vi "简易计算器.vi"() -> ()   [LabVIEW 2018]
panel:
  out "布尔":bool
  out "字符串 3":string
  out "结果":dbl
  out "数字":dbl
  out "字符串 2":string
  out "字符串":string
  in  "簇":T1
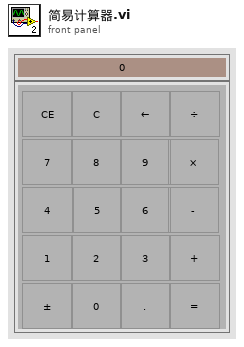
[diagram p1: front panel]
types:
  T1 = cluster{"确定按钮":bool, "确定按钮 2":bool, "确定按钮 3":bool, "确定按钮 4":bool, "确定按钮 5":bool, "确定按钮 6":bool, "确定按钮 7":bool, "确定按钮 8":bool, "确定按钮 9":bool, "确定按钮 10":bool, "确定按钮 17":bool, "确定按钮 18":bool, "确定按钮 19":bool, "确定按钮 20":bool, "确定按钮 16":bool, "确定按钮 15":bool, "确定按钮 14":bool, "确定按钮 13":bool, "确定按钮 12":bool, "确定按钮 11":bool}
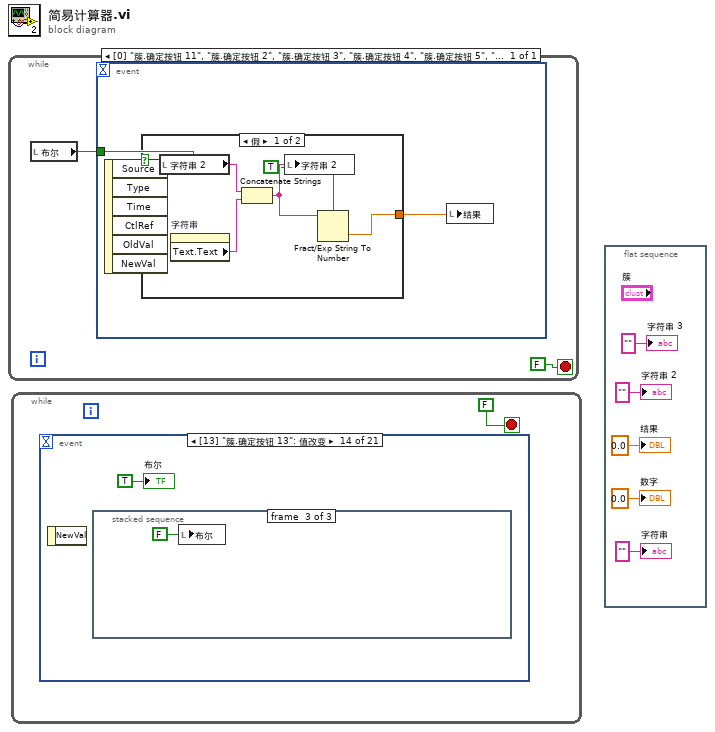
[diagram p0: block diagram]
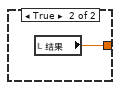
[diagram p2: hidden frame]
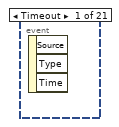
[diagram p3: hidden frame]
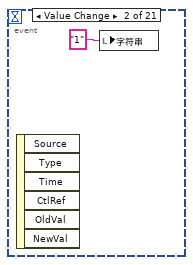
[diagram p4: hidden frame]
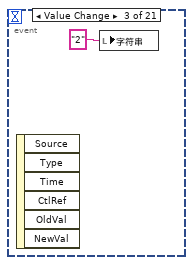
[diagram p5: hidden frame]
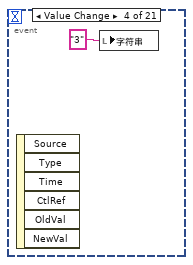
[diagram p6: hidden frame]
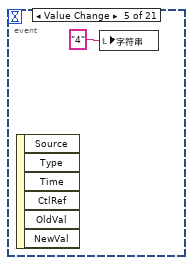
[diagram p7: hidden frame]
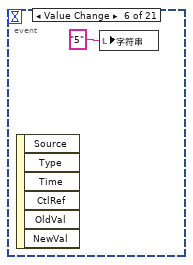
[diagram p8: hidden frame]
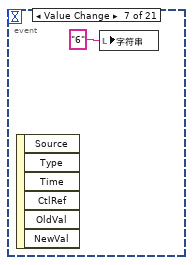
[diagram p9: hidden frame]
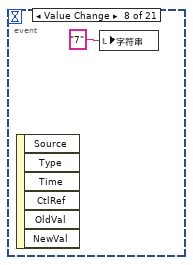
[diagram p10: hidden frame]
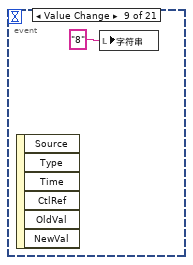
[diagram p11: hidden frame]
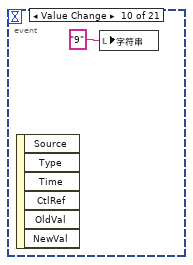
[diagram p12: hidden frame]
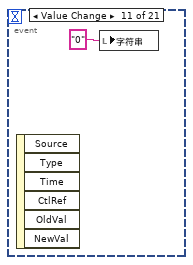
[diagram p13: hidden frame]
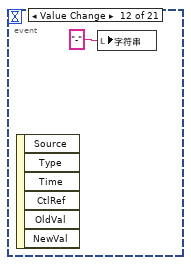
[diagram p14: hidden frame]
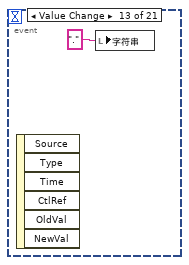
[diagram p15: hidden frame]
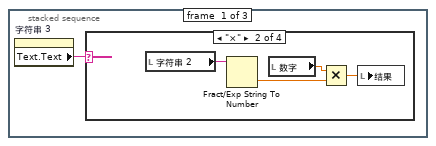
[diagram p16: hidden frame]
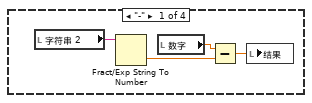
[diagram p17: hidden frame]
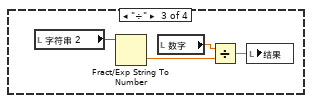
[diagram p18: hidden frame]
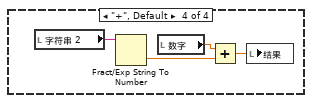
[diagram p19: hidden frame]
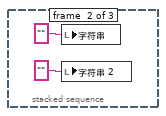
[diagram p20: hidden frame]
diagram:
  n1 = while {
    stop <- FALSE stop-if-true
    n2 = local read "布尔"() -> (w1:bool)
    n3 = event shown="[0] \"簇.确定按钮 11\", \"簇.确定按钮 2\", \"簇.确定按钮 3\", \"簇.确定按钮 4\", \"簇.确定按钮 5\", \"簇.确定按钮 6\", \"簇.确定按钮 7\", \"簇.确定按钮 8\", \"簇.确定按钮 9\", \"簇.确定按钮 10\", \"簇.确定按钮 12\", \"簇.确定按钮\": 值改变" {
      selector: _ -> [_]
      dyn-events: _ -> [_]
      timeout: _ -> [_]
      tunnel: w1 -> [w3]
      event "簇.确定按钮 11", "簇.确定按钮 2", "簇.确定按钮 3", "簇.确定按钮 4", "簇.确定按钮 5", "簇.确定按钮 6", "簇.确定按钮 7", "簇.确定按钮 8", "簇.确定按钮 9", "簇.确定按钮 10", "簇.确定按钮 12", "簇.确定按钮": Value Change {
        n4 = event-data() -> ()  [unwired: 1 in, 6 out]
        n5 = case shown="假" w3 {
          tunnel: [w7 w10] -> w4
          frame False {
            n6 = local read "字符串 2"() -> (w9:string)
            n7 = property on="字符串" class="Str"() -> ("Text.Text"=w6:string)  [unwired: 2 in, 2 out]
            n8 = Concatenate Strings(w9, w6) -> (w8:string)
            n9 = local write "字符串 2"(w8) -> ()
            n10 = Fract/Exp String To Number(use system decimal point (T)=TRUE ("使用系统小数点(T)"), string=w8) -> (number=w7:dbl)  [unwired: 2 in, 1 out]
          }
          frame True {
            n11 = local read "结果"() -> (w10:dbl)
          }
        }
        n12 = local write "结果"(w4) -> ()
      }
    }
  }
  n13 = while {
    stop <- FALSE stop-if-true
    n14 = event shown="[13] \"簇.确定按钮 13\": 值改变" {
      selector: _ -> [_ _ _ _ _ _ _ _ _ _ _ _ _ _ _ _ _ _ _ _ _]
      dyn-events: _ -> [_ _ _ _ _ _ _ _ _ _ _ _ _ _ _ _ _ _ _ _ _]
      timeout: _ -> [_ _ _ _ _ _ _ _ _ _ _ _ _ _ _ _ _ _ _ _ _]
      event Timeout {
        n15 = event-data() -> ()  [unwired: 1 in, 3 out]
      }
      event "簇.确定按钮": Value Change {
        n16 = event-data() -> ()  [unwired: 1 in, 6 out]
        n17 = local write "字符串"("1" ("字符串")) -> ()
      }
      event "簇.确定按钮 2": Value Change {
        n18 = event-data() -> ()  [unwired: 1 in, 6 out]
        n19 = local write "字符串"("2" ("字符串")) -> ()
      }
      event "簇.确定按钮 3": Value Change {
        n20 = event-data() -> ()  [unwired: 1 in, 6 out]
        n21 = local write "字符串"("3" ("字符串")) -> ()
      }
      event "簇.确定按钮 4": Value Change {
        n22 = event-data() -> ()  [unwired: 1 in, 6 out]
        n23 = local write "字符串"("4" ("字符串")) -> ()
      }
      event "簇.确定按钮 5": Value Change {
        n24 = event-data() -> ()  [unwired: 1 in, 6 out]
        n25 = local write "字符串"("5" ("字符串")) -> ()
      }
      event "簇.确定按钮 6": Value Change {
        n26 = event-data() -> ()  [unwired: 1 in, 6 out]
        n27 = local write "字符串"("6" ("字符串")) -> ()
      }
      event "簇.确定按钮 7": Value Change {
        n28 = event-data() -> ()  [unwired: 1 in, 6 out]
        n29 = local write "字符串"("7" ("字符串")) -> ()
      }
      event "簇.确定按钮 8": Value Change {
        n30 = event-data() -> ()  [unwired: 1 in, 6 out]
        n31 = local write "字符串"("8" ("字符串")) -> ()
      }
      event "簇.确定按钮 9": Value Change {
        n32 = event-data() -> ()  [unwired: 1 in, 6 out]
        n33 = local write "字符串"("9" ("字符串")) -> ()
      }
      event "簇.确定按钮 10": Value Change {
        n34 = event-data() -> ()  [unwired: 1 in, 6 out]
        n35 = local write "字符串"("0" ("字符串")) -> ()
      }
      event "簇.确定按钮 11": Value Change {
        n36 = event-data() -> ()  [unwired: 1 in, 6 out]
        n37 = local write "字符串"("-" ("字符串")) -> ()
      }
      event "簇.确定按钮 12": Value Change {
        n38 = event-data() -> ()  [unwired: 1 in, 6 out]
        n39 = local write "字符串"("." ("字符串")) -> ()
      }
      event "簇.确定按钮 13": Value Change {
        n40 = event-data() -> ()  [unwired: 1 in, 1 out]
        n41 = stacked-sequence {
          frame #0 {
            n42 = property on="字符串 3" class="Str"() -> ("Text.Text"=w25:string)  [unwired: 2 in, 2 out]
            n43 = case shown="\"×\"" w25 {
              frame "-" {
                n44 = local read "字符串 2"() -> (w26:string)
                n45 = Fract/Exp String To Number(string=w26) -> (number=w29:dbl)  [unwired: 3 in, 1 out]
                n46 = local read "数字"() -> (w28:dbl)
                n47 = Subtract(x=w28, y=w29) -> (x-y=w27:dbl)
                n48 = local write "结果"(w27) -> ()
              }
              frame "×" {
                n49 = local read "字符串 2"() -> (w30:string)
                n50 = Fract/Exp String To Number(string=w30) -> (number=w33:dbl)  [unwired: 3 in, 1 out]
                n51 = local read "数字"() -> (w32:dbl)
                n52 = Multiply(x=w32, y=w33) -> (x*y=w31:dbl)
                n53 = local write "结果"(w31) -> ()
              }
              frame "÷" {
                n54 = local read "字符串 2"() -> (w34:string)
                n55 = Fract/Exp String To Number(string=w34) -> (number=w37:dbl)  [unwired: 3 in, 1 out]
                n56 = local read "数字"() -> (w36:dbl)
                n57 = Divide(x=w36, y=w37) -> (x/y=w35:dbl)
                n58 = local write "结果"(w35) -> ()
              }
              frame "+", Default {
                n59 = local read "字符串 2"() -> (w40:string)
                n60 = Fract/Exp String To Number(string=w40) -> (number=w39:dbl)  [unwired: 3 in, 1 out]
                n61 = local read "数字"() -> (w41:dbl)
                n62 = Add(x=w41, y=w39) -> (x+y=w38:dbl)
                n63 = local write "结果"(w38) -> ()
              }
            }
          }
          frame #1 {
            n64 = local write "字符串"("" ("字符串")) -> ()
            n65 = local write "字符串 2"("" ("字符串 2")) -> ()
          }
          frame #2 {
            n66 = local write "布尔"(FALSE ("布尔")) -> ()
          }
        }
        "布尔" <- TRUE ("布尔")
      }
      event "簇.确定按钮 14": Value Change {
        n67 = event-data() -> ()  [unwired: 1 in, 6 out]
        n68 = stacked-sequence {
          frame #0 {
            n69 = local read "字符串 2"() -> (w47:string)
            n70 = Fract/Exp String To Number(string=w47) -> (number=w46:dbl)  [unwired: 3 in, 1 out]
            n71 = local write "数字"(w46) -> ()
          }
          frame #1 {
            n72 = local write "字符串"("" ("字符串")) -> ()
            n73 = local write "字符串 2"("" ("字符串 2")) -> ()
          }
        }
        n74 = local write "字符串 3"("+" ("字符串")) -> ()
      }
      event "簇.确定按钮 15": Value Change {
        n75 = event-data() -> ()  [unwired: 1 in, 6 out]
        n76 = stacked-sequence {
          frame #0 {
            n77 = local read "字符串 2"() -> (w52:string)
            n78 = Fract/Exp String To Number(string=w52) -> (number=w51:dbl)  [unwired: 3 in, 1 out]
            n79 = local write "数字"(w51) -> ()
          }
          frame #1 {
            n80 = local write "字符串"("" ("字符串")) -> ()
            n81 = local write "字符串 2"("" ("字符串 2")) -> ()
          }
        }
        n82 = local write "字符串 3"("-" ("字符串")) -> ()
      }
      event "簇.确定按钮 16": Value Change {
        n83 = event-data() -> ()  [unwired: 1 in, 6 out]
        n84 = stacked-sequence {
          frame #0 {
            n85 = local read "字符串 2"() -> (w57:string)
            n86 = Fract/Exp String To Number(string=w57) -> (number=w56:dbl)  [unwired: 3 in, 1 out]
            n87 = local write "数字"(w56) -> ()
          }
          frame #1 {
            n88 = local write "字符串"("" ("字符串")) -> ()
            n89 = local write "字符串 2"("" ("字符串 2")) -> ()
          }
        }
        n90 = local write "字符串 3"("×" ("字符串")) -> ()
      }
      event "簇.确定按钮 17": Value Change {
        n91 = event-data() -> ()  [unwired: 1 in, 6 out]
        n92 = local write "字符串 2"("" ("字符串 2")) -> ()
        n93 = local write "结果"(0.0 ("结果")) -> ()
      }
      event "簇.确定按钮 18": Value Change {
        n94 = event-data() -> ()  [unwired: 1 in, 6 out]
        n95 = local write "字符串 3"("" ("字符串 3")) -> ()
        n96 = local write "字符串 2"("" ("字符串 2")) -> ()
        n97 = local write "结果"(0.0 ("结果")) -> ()
        n98 = local write "数字"(0.0 ("数字")) -> ()
        n99 = local write "字符串"("" ("字符串")) -> ()
      }
      event "簇.确定按钮 19": Value Change {
        n100 = event-data() -> ()  [unwired: 1 in, 6 out]
        n101 = local read "字符串 2"() -> (w69:string)
        n102 = String Length(string=w69) -> (length=w71:i32)
        n103 = Decrement(x=w71) -> (x-1=w70:i32)
        n104 = String Subset(string=w69, length (rest)=w70) -> (substring=w67:string)  [unwired: 1 in]
        n105 = Fract/Exp String To Number(string=w67) -> (number=w68:dbl)  [unwired: 3 in, 1 out]
        n106 = local write "字符串 2"(w67) -> ()
        n107 = local write "结果"(w68) -> ()
      }
      event "簇.确定按钮 20": Value Change {
        n108 = event-data() -> ()  [unwired: 1 in, 6 out]
        n109 = stacked-sequence {
          frame #0 {
            n110 = local read "字符串 2"() -> (w74:string)
            n111 = Fract/Exp String To Number(string=w74) -> (number=w73:dbl)  [unwired: 3 in, 1 out]
            n112 = local write "数字"(w73) -> ()
          }
          frame #1 {
            n113 = local write "字符串"("" ("字符串")) -> ()
            n114 = local write "字符串 2"("" ("字符串 2")) -> ()
          }
        }
        n115 = local write "字符串 3"("÷" ("字符串")) -> ()
      }
    }
  }
  n116 = flat-sequence {
    frame #0 {
      "数字" <- 0.0 ("数字 2")
      "结果" <- 0.0 ("结果")
      "字符串 2" <- "" ("字符串")
      "字符串 3" <- "" ("字符串 3")
      "字符串" <- "" ("字符串 2")
    }
  }
